vi "ZhiYuan ZDS Series for TCP Acquire Multiple Waveforms.vi"() -> ()   [LabVIEW 2015]
doc: "This example shows how to configure multiple channels and acquire waveforms from multiple channels."
uses:
  ZhiYuan ZDS Series for TCP.lvlib
  Public/Data/Read Waveform (Multiple).vi
panel:
  in  "Scale(H)":T1(ring)=enum."10us"
  in  "Offset (H)":dbl
  in  "Probe(B)":i32(ring)=12 items=["0.001", "0.002", "0.005", "0.01", "0.02", "0.05", "0.1", "0.2", "0.5", "1", "2", "5", "10", "20", "50", "100", "200", "500", "1000"]
  in  "Scale(B)":dbl=0.5 caption="Scale" min=0.0 format="%#_13g"
  in  "Offset(B)":dbl=-1.4 format="%#_13g"
  in  "Probe(A)":i32(ring)=12 items=["0.001", "0.002", "0.005", "0.01", "0.02", "0.05", "0.1", "0.2", "0.5", "1", "2", "5", "10", "20", "50", "100", "200", "500", "1000"]
  in  "Scale(A)":dbl=0.5 caption="Scale" min=0.0 format="%#_13g"
  in  "Offset(A)":dbl=-1.4 format="%#_13g"
  in  "Maximum Time (ms)":u32=5000
  in  "Vertical Coupling(B)":i32(ring)=1 items=["AC", "DC", "Ground"]
  in  "Channel B":i32(ring)=2 items=["Channel 1"=1, "Channel 2"=2, "Channel 3"=3, "Channel 4"=4]
  in  "Vertical Coupling(A)":i32(ring)=1 items=["AC", "DC", "Ground"]
  in  "Channel  A":i32(ring)=1 items=["Channel 1"=1, "Channel 2"=2, "Channel 3"=3, "Channel 4"=4]
  out "Waveform Data":dbl[][](graph)
  in  "VISA resource name":refnum<visa-resource-name>
  # "(c) 2012 National Instruments.  ALL RIGHTS RESERVED."
  # "Channel A"
  # "Channel B"
  # "Horizontal"
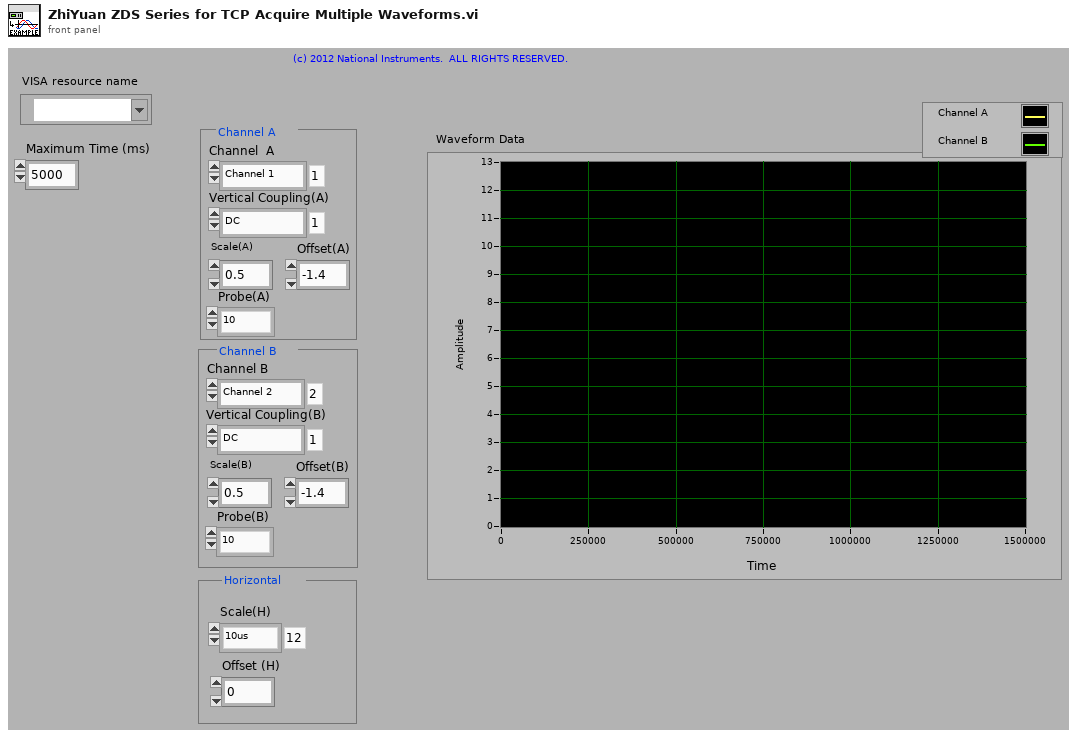
[diagram p1: front panel]
types:
  T1 = enum16{"1ns", "2ns", "5ns", "10ns", "20ns", "50ns", "100ns", "200ns", "500ns", "1us", "2us", "5us", "10us", "20us", "50us", "100us", "200us", "500us", "1ms", "2ms", "5ms", "10ms", "20ms", "50ms", "100ms", "200ms", "500ms", "1s", "2s", "5s", "10s", "20s", "50s", "100s"}
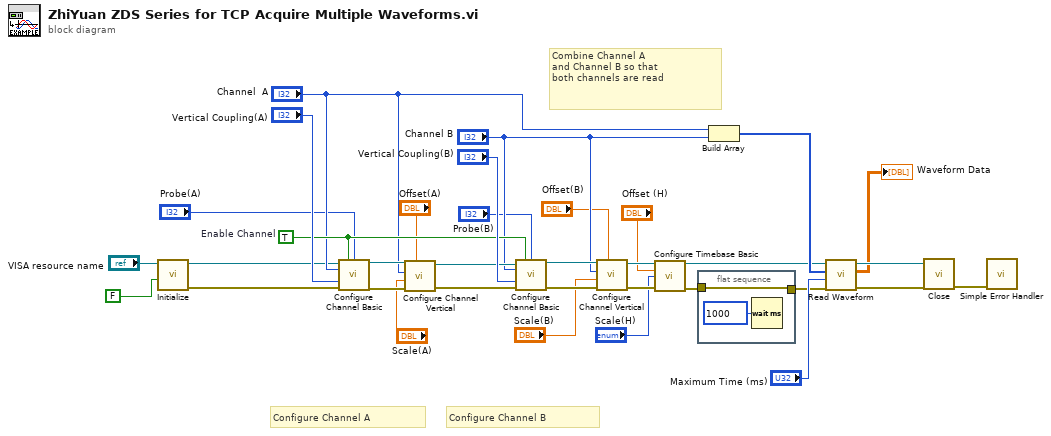
[diagram p0: block diagram]
diagram:
  w25 = TRUE  # Enable Channel
  # "Combine Channel A\nand Channel B so that\nboth channels are read"
  # "Configure Channel B"
  # "Configure Channel A"
  n1 = call "Initialize.vi"("Reset (True)"=FALSE, "VISA resource name"="VISA resource name") -> ("error out"=w7:errorcluster, "VISA resource name out"=w8:refnum<visa-resource-name>)  [unwired: 8 in]
  n2 = call "Configure Channel Basic.vi"("VISA resource name"=w8, "Enable Channel (F: Disable)"=w25, "Probe"="Probe(A)", "Channel (1: Channel 1)"="Channel  A", "Coupling Mode (1: DC)"="Vertical Coupling(A)", "error in (no error)"=w7) -> ("VISA resource name out"=w24:refnum<visa-resource-name>, "error out"=w21:errorcluster)  [unwired: 8 in]
  n3 = call "Configure Channel Vertical.vi"("Offset (0)"="Offset(A)", "error in (no error)"=w21, "Scale (1)"="Scale(A)", "Channel (1: Channel 1)"="Channel  A", "VISA resource name"=w24) -> ("error out"=w22:errorcluster, "VISA resource name out"=w23:refnum<visa-resource-name>)  [unwired: 5 in]
  n4 = call "Configure Channel Basic.vi"("VISA resource name"=w23, "Enable Channel (F: Disable)"=w25, "Probe"="Probe(B)", "Channel (1: Channel 1)"="Channel B", "Coupling Mode (1: DC)"="Vertical Coupling(B)", "error in (no error)"=w22) -> ("VISA resource name out"=w19:refnum<visa-resource-name>, "error out"=w18:errorcluster)  [unwired: 8 in]
  n5 = call "Configure Channel Vertical.vi"("Offset (0)"="Offset(B)", "error in (no error)"=w18, "Scale (1)"="Scale(B)", "Channel (1: Channel 1)"="Channel B", "VISA resource name"=w19) -> ("error out"=w12:errorcluster, "VISA resource name out"=w13:refnum<visa-resource-name>)  [unwired: 5 in]
  n6 = call "Configure Timebase Basic.vi"("VISA resource name"=w13, "Offset (0)"="Offset (H)", "Scale"="Scale(H)", "error in (no error)"=w12) -> ("VISA resource name out"=w11:refnum<visa-resource-name>, "error out"=w10:errorcluster)  [unwired: 10 in]
  n7 = flat-sequence {
    tunnel: [w36] -> w14
    tunnel: w10 -> [w36]
    frame #0 {
      n8 = Wait (ms)(milliseconds to wait=u32 1000) -> ()  [unwired: 1 out]
    }
  }
  n9 = Build Array("Channel  A", "Channel B") -> (w28:i32[])
  n10 = call-poly "Read Waveform.vi"("error in (no error)"=w14, "Maximum Time (5000 ms)"="Maximum Time (ms)", "Channels"=w28, "VISA resource name"=w11) -> ("error out"=w30:errorcluster, "Waveform Data"=→"Waveform Data":dbl[][], "VISA resource name out"=w32:refnum<visa-resource-name>)  [unwired: 5 in]
  n11 = call "Close.vi"("error in (no error)"=w30, "VISA resource name"=w32) -> ("error out"=w33:errorcluster)  [unwired: 9 in]
  n12 = call <vilib>:"Simple Error Handler.vi"("error in (no error)"=w33) -> ()  [unwired: 4 in, 5 out]
